vi "Total数据写入.vi"(6 "Total数值":string, 9 "configuration file path":path caption="配置文件的路径") -> ()   [LabVIEW 2011]
uses:
  <vilib>/Utility/config.llb/NI_LVConfig.lvlib
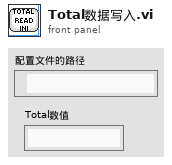
[diagram p1: front panel]
types:
  T1 = typedef "NI_LVConfig.lvlib/Config Data RefNum.ctl" = refnum<k1>
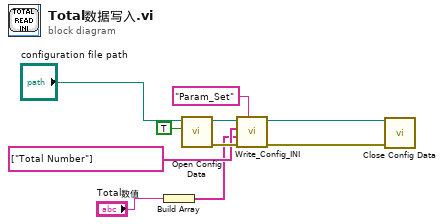
[diagram p0: block diagram]
diagram:
  n1 = Build Array("Total数值") -> (w1:string[])
  n2 = call <vilib>:"Open Config Data.vi"("create file if necessary (T)"=TRUE, "configuration file path"="configuration file path") -> ("error out"=w7:errorcluster, "refnum"=w8:T1)  [unwired: 7 in, 1 out]
  n3 = call "Write_Config_INI.vi"("section"="Param_Set", "error in (no error)"=w7, "Inputs"=w1, "Keys"=string[] ["Total Number"], "refnum"=w8) -> ("error out"=w4:errorcluster, "refnum 2"=w5:T1)  [unwired: 5 in]
  n4 = call <vilib>:"Close Config Data.vi"("error in (no error)"=w4, "refnum"=w5) -> ()  [unwired: 8 in, 2 out]
